vi "Load Pre-Index.vi"(8 "error in":errorcluster) -> (0 "error out":errorcluster)   [LabVIEW 2020]
uses:
  <vilib>/regexp/Match Regular Expression.xnode
  DBMap/DBMap.lvclass
  DBSet/DBSet.lvclass
  <vilib>/zip/NI_Unzip.lvlib
panel:
  out "Status":string
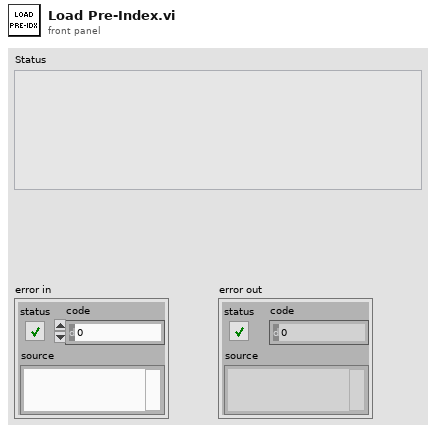
[diagram p1: front panel]
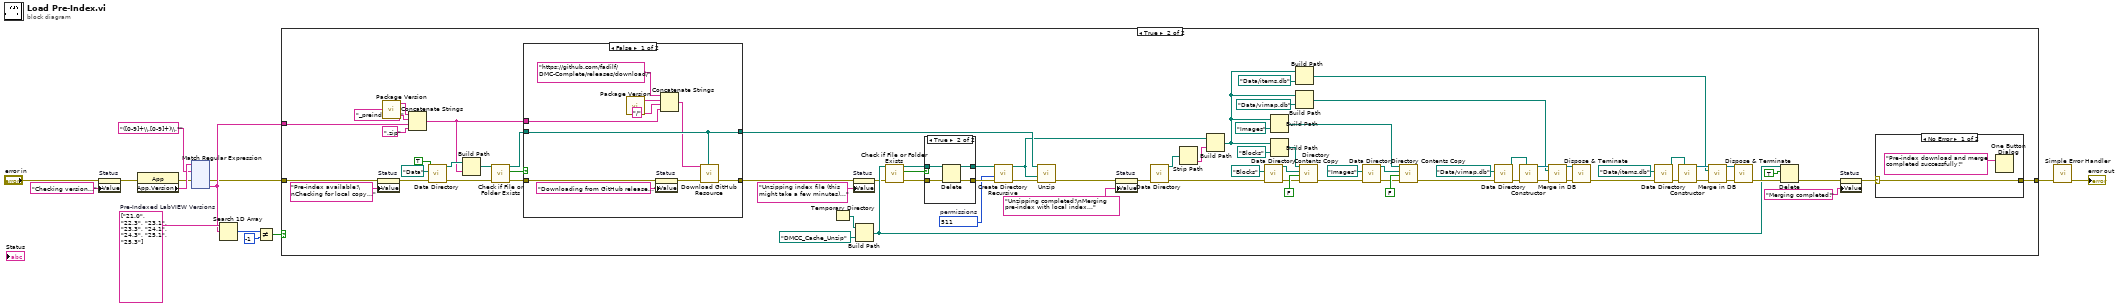
[diagram p0: block diagram]
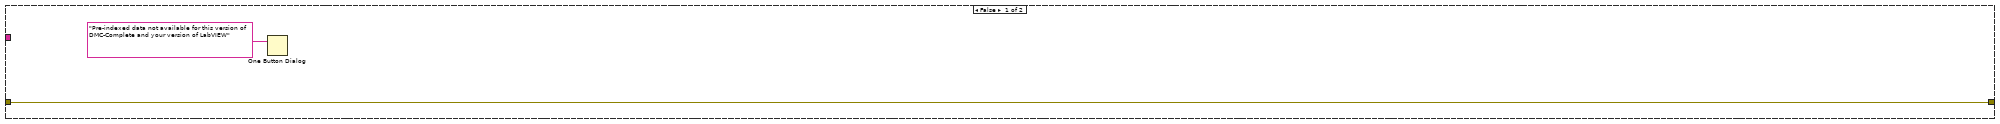
[diagram p2: hidden frame]
diagram:
  w12 = string[] ["21.0", "22.3", "23.1", "23.3", "24.1", "24.3", "25.1", "25.3"]  # Pre-Indexed LabVIEW Versions
  n1 = property on="Status" class="Str"(error in="error in", "Value"="Checking version..." ("Status")) -> (error out=w2:errorcluster)  [unwired: 1 in, 1 out]
  n2 = property class="App"(error in=w2) -> (error out=w8:errorcluster, "App.Version"=w14:string)  [unwired: 1 in, 1 out]
  n3 = xnode "Match Regular Expression"("input string"=w14, "regular expression"="([0-9]+\\.[0-9]+)\\.*", "error in"=w8) -> ("error out"=w7:errorcluster, "submatch 1"=w9:string)  [unwired: 3 in, 4 out]
  n4 = Search 1D Array(1D array=w12, element=w9) -> (index of element=w11:i32)  [unwired: 1 in]
  n5 = Not Equal?(x=w11, y=-1) -> (x != y?=w6:bool)
  n6 = case shown="True" w6 {
    tunnel: w9 -> [_ w91]
    tunnel: w7 -> [w15 w29]
    tunnel: [w15 w17] -> w5
    frame False {
      n7 = One Button Dialog(message="Pre-indexed data not available for this version of DMC-Complete and your version of LabVIEW") -> ()  [unwired: 1 in, 1 out]
    }
    frame True {
      w40 = i16 511  # permissions
      n8 = property on="Status" class="Str"(error in=w29, "Value"="Pre-index available!\nChecking for local copy..." ("Status")) -> (error out=w28:errorcluster)  [unwired: 1 in, 1 out]
      n9 = call "Package Version.vi"() -> ("Package Version"=w89:string)  [unwired: 2 in]
      n10 = Concatenate Strings(w89, "_preindexed_" ("string"), w91, ".zip" ("string")) -> (w74:string)
      n11 = call "Data Directory.vi"("error in (no error)"=w28, "Subdirectory"=path "Data" ("base path"), "Create if doesn't exist? (F)"=TRUE) -> ("error out"=w27:errorcluster, "Data directory"=w75:path)  [unwired: 7 in]
      n12 = Build Path(base path=w75, name or relative path=w74) -> (appended path=w73:path)
      n13 = call <vilib>:"Check if File or Folder Exists.vi"("error in (no error)"=w27, "path"=w73) -> ("error out"=w87:errorcluster, "file or folder exists?"=w88:bool, "dup path"=w86:path)  [unwired: 7 in]
      n14 = case shown="False" w88 {
        tunnel: w87 -> [w106 w112]
        tunnel: w74 -> [w109 _]
        tunnel: w86 -> [w105 w113]
        tunnel: [w102 w112] -> w25
        tunnel: [w105 w113] -> w85
        frame False {
          n15 = call "Package Version.vi"() -> ("Package Version"=w110:string)  [unwired: 2 in]
          n16 = property on="Status" class="Str"(error in=w106, "Value"="Downloading from GitHub release..." ("Status")) -> (error out=w103:errorcluster)  [unwired: 1 in, 1 out]
          n17 = Concatenate Strings("https://github.com/fadilf/DMC-Complete/releases/download/", w110, "/" ("string"), w109) -> (w104:string)
          n18 = call "Download GitHub Resource.vi"("Output file"=w105, "error in (no error)"=w103, "URL"=w104) -> ("error out"=w102:errorcluster)  [unwired: 8 in]
        }
        frame True {
        }
      }
      n19 = Temporary Directory() -> (w84:path)
      n20 = property on="Status" class="Str"(error in=w25, "Value"="Unzipping index file (this might take a few minutes)..." ("Status")) -> (error out=w24:errorcluster)  [unwired: 1 in, 1 out]
      n21 = Build Path(base path=w84, name or relative path=path "DMCC_Cache_Unzip") -> (appended path=w45:path)
      n22 = call <vilib>:"Check if File or Folder Exists.vi"("error in (no error)"=w24, "path"=w45) -> ("error out"=w82:errorcluster, "file or folder exists?"=w81:bool)  [unwired: 7 in, 1 out]
      n23 = case shown="True" w81 {
        tunnel: [w97 w101] -> w42
        tunnel: [w96 w100] -> w43
        tunnel: w82 -> [w97 w99]
        tunnel: w45 -> [w96 w98]
        frame False {
        }
        frame True {
          n24 = Delete(path (use dialog)=w98, error in=w99) -> (deleted path=w100:path, error out=w101:errorcluster)  [unwired: 3 in, 1 out]
        }
      }
      n25 = call <vilib>:"Create Directory Recursive.vi"("error in (no error)"=w42, "permissions"=w40, "directory"=w43) -> ("error out"=w41:errorcluster, "directory copy"=w80:path)  [unwired: 2 in, 1 out]
      n26 = call <vilib>:"Unzip.vi"("error in (no error)"=w41, "Target directory (same as Zip file if empty)"=w80, "Zip file"=w85) -> ("error out"=w22:errorcluster)  [unwired: 6 in, 2 out]
      n27 = property on="Status" class="Str"(error in=w22, "Value"="Unzipping completed!\nMerging pre-index with local index..." ("Status")) -> (error out=w21:errorcluster)  [unwired: 1 in, 1 out]
      n28 = call "Data Directory.vi"("error in (no error)"=w21) -> ("error out"=w72:errorcluster, "Data directory"=w70:path)  [unwired: 9 in]
      n29 = Strip Path(path=w70) -> (name=w79:string)  [unwired: 1 out]
      n30 = Build Path(base path=w80, name or relative path=w79) -> (appended path=w62:path)
      n31 = call "Data Directory.vi"("error in (no error)"=w72, "Subdirectory"=path "Blocks") -> ("error out"=w37:errorcluster, "Data directory"=w31:path)  [unwired: 8 in]
      n32 = Build Path(base path=w62, name or relative path=path "Images") -> (appended path=w68:path)
      n33 = Build Path(base path=w62, name or relative path=path "Blocks") -> (appended path=w71:path)
      n34 = Build Path(base path=w62, name or relative path=path "Data/items.db") -> (appended path=w47:path)
      n35 = Build Path(base path=w62, name or relative path=path "Data/vimap.db") -> (appended path=w56:path)
      n36 = call "Directory Contents Copy.vi"("error in"=w37, "overwrite (F)"=FALSE, "Destination Folder"=w31, "Source Folder"=w71) -> ("error out"=w34:errorcluster)  [unwired: 7 in]
      n37 = call "Data Directory.vi"("error in (no error)"=w34, "Subdirectory"=path "Images") -> ("error out"=w33:errorcluster, "Data directory"=w32:path)  [unwired: 8 in]
      n38 = call "Directory Contents Copy.vi"("error in"=w33, "overwrite (F)"=FALSE, "Destination Folder"=w32, "Source Folder"=w68) -> ("error out"=w61:errorcluster)  [unwired: 7 in]
      n39 = call "Data Directory.vi"("error in (no error)"=w61, "Subdirectory"=path "Data/vimap.db" ("name or relative path")) -> ("error out"=w66:errorcluster, "Data directory"=w65:path)  [unwired: 8 in]
      n40 = call "Constructor.vi"("SQLite DB Path"=w65, "error in (no error)"=w66) -> ("error out"=w60:errorcluster, "DBMap out"=w58:refnum<class "DBMap.lvclass">)  [unwired: 8 in]
      n41 = call "Merge in DB.vi"("DBMap in"=w58, "SQLite DB Path"=w56, "error in (no error)"=w60) -> ("DBMap out"=w57:refnum<class "DBMap.lvclass">, "error out"=w59:errorcluster)  [unwired: 11 in]
      n42 = call-dynamic "Dispose & Teminate.vi"("DBMap in"=w57, "error in (no error)"=w59) -> ("error out"=w52:errorcluster)  [unwired: 12 in, 1 out]
      n43 = call "Data Directory.vi"("error in (no error)"=w52, "Subdirectory"=path "Data/items.db" ("name or relative path")) -> ("error out"=w54:errorcluster, "Data directory"=w55:path)  [unwired: 8 in]
      n44 = call "Constructor.vi"("SQLite DB Path"=w55, "error in (no error)"=w54) -> ("DBSet out"=w49:refnum<class "DBSet.lvclass">, "error out"=w51:errorcluster)  [unwired: 12 in]
      n45 = call "Merge in DB.vi"("DBSet in"=w49, "SQLite DB Path"=w47, "error in (no error)"=w51) -> ("DBSet out"=w48:refnum<class "DBSet.lvclass">, "error out"=w50:errorcluster)  [unwired: 11 in]
      n46 = call-dynamic "Dispose & Terminate.vi"("DBSet in"=w48, "error in (no error)"=w50) -> ("error out"=w46:errorcluster)  [unwired: 12 in, 1 out]
      n47 = Delete(path (use dialog)=w45, entire hierarchy (F)=TRUE, error in=w46) -> (error out=w19:errorcluster)  [unwired: 2 in, 2 out]
      n48 = property on="Status" class="Str"(error in=w19, "Value"="Merging completed!" ("Status")) -> (error out=w18:errorcluster)  [unwired: 1 in, 1 out]
      n49 = case shown="No Error" w18 {
        selector: w18 -> [w93 w95]
        tunnel: [w93 w95] -> w17
        frame No Error {
          n50 = One Button Dialog(message="Pre-index download and merge completed successfully!") -> ()  [unwired: 1 in, 1 out]
        }
        frame Error {
        }
      }
    }
  }
  n51 = call <vilib>:"Simple Error Handler.vi"("error in (no error)"=w5) -> ("error out"=→"error out":errorcluster)  [unwired: 4 in, 4 out]
